vi "Read Config.vi"(8 "error in (no error)":errorcluster, 10 "Resource In":variant, 11 "Analyze Parameter ROI in":refnum<class "Analyze Parameter ROI.lvclass">) -> (0 "error out":errorcluster, 2 "Resource Out":variant, 3 "Analyze Parameter ROI out":refnum<class "Analyze Parameter ROI.lvclass">)   [LabVIEW 2014, in "Analyze Parameter ROI.lvclass"]
uses:
  Analyze Parameter ROI.lvclass
  <vilib>/Utility/config.llb/Config Data RefNum.ctl
  Analyze Parameter ROI.lvclass/Analyze Parameter ROI.ctl
  <vilib>/Utility/config.llb/NI_LVConfig.lvlib
  Utility/POLARIS Vision utility.lvlib
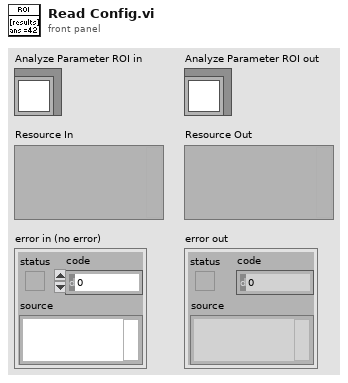
[diagram p1: front panel]
types:
  T1 = typedef "NI_LVConfig.lvlib/Config Data RefNum.ctl" = refnum<k1>
  T2 = typedef "ROI Descriptor" = cluster{"Global Rectangle":i32[], "Contours":cluster{"ID":enum32{"External", "Internal"}, "Type":u32, "Coordinates":i32[]}[]}
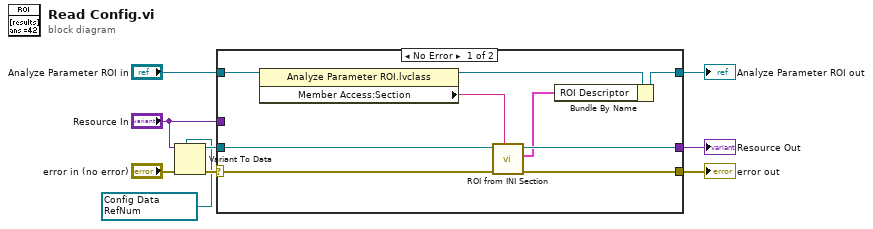
[diagram p0: block diagram]
diagram:
  w1 = T1 refnum items=["config data"] ("refnum")
  n1 = Variant To Data(error in="error in (no error)", type=w1, Variant="Resource In") -> (data=w9:T1, error out=w8:errorcluster)
  n2 = case shown="No Error" w8 {
    selector: w8 -> [w13 w20]
    tunnel: w9 -> [w14 _]
    tunnel: "Analyze Parameter ROI in" -> [w16 w19]
    tunnel: [w18 w19] -> w4
    tunnel: [w12 w21] -> w3
    tunnel: [w11 w20] -> w2
    tunnel: "Resource In" -> [_ w21]
    frame No Error {
      n3 = property class="Analyze Parameter ROI.lvclass"(reference=w16) -> (reference out=w17:refnum<class "Analyze Parameter ROI.lvclass">, "Member Access:Section"=w15:string)  [unwired: 1 in, 1 out]
      n4 = call "ROI from INI Section.vi"("section"=w15, "error in (no error)"=w13, "refnum in"=w14) -> ("error out"=w11:errorcluster, "ROI"=w10:T2, "refnum out"=w12:T1)  [unwired: 6 in]
      n5 = Bundle By Name(cluster=w17, "ROI Descriptor"=w10) -> (w18:refnum<class "Analyze Parameter ROI.lvclass">)
    }
    frame Error {
    }
  }
  "error out" <- w2
  "Analyze Parameter ROI out" <- w4
  "Resource Out" <- w3
